vi "UDT_admittanceLibrary_selectData.vi"() -> (3 "Unit Test Framework Results":T1)   [LabVIEW 2017]
doc: "Use this template to create a user-defined test VI. Define your test requirements and wire the results to the <b>Result (Test)</b> control. Do not modify the <b>Unit Test Framework Results</b> indicator."
uses:
  <vilib>/utf/common/utf_test_result_troll.ctl
  <vilib>/utf/common/utf_test_result.ctl
  <vilib>/utf/common/utf_test_result_failure.ctl
  <vilib>/utf/common/utf_test_comparison_operators.ctl
  <vilib>/utf/common/utf_vi_tag.ctl
  RT/TypeDefs/allData.ctl
  RT/TypeDefs/dataOut.ctl
  RT/TypeDefs/dataIn.ctl
  <vilib>/Control Software Solutions Ltd/UTF Helper/SubVIs/UTF Double Equals.vi
  <vilib>/Control Software Solutions Ltd/UTF Helper/SubVIs/UTF Boolean Equals.vi
  RT/Admittance Controller/admittanceControllerLibrary.lvlib
  <vilib>/Control Software Solutions Ltd/UTF Helper/Unit Test Helper.lvlib
  <vilib>/utf/NI_UnitTestFramework.lvlib
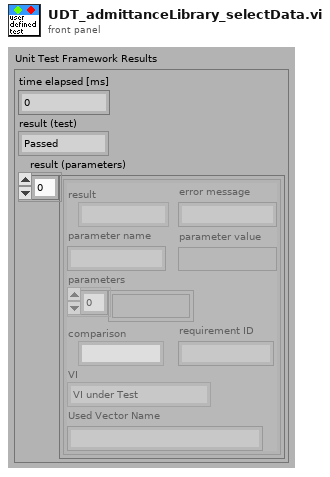
[diagram p1: front panel]
types:
  T1 = typedef "NI_UnitTestFramework.lvlib/utf_test_result_troll.ctl" = cluster{"time elapsed [ms]":u32, "result (test)":T2, "result (parameters)":T3[]}
  T2 = typedef "NI_UnitTestFramework.lvlib/utf_test_result.ctl" = enum16{"Passed", "Failed", "Error", "Skipped", "Not Processed"}
  T3 = typedef "NI_UnitTestFramework.lvlib/utf_test_result_failure.ctl" = cluster{"result":T2, "error message":string, "parameter name":string, "parameter value":variant, "parameters":variant[], "comparison":T4, "requirement ID":string, "VI":T5, "Used Vector Name":string}
  T4 = typedef "NI_UnitTestFramework.lvlib/utf_test_comparison_operators.ctl" = enum16{"=", "!=", ">", ">=", "<", "<=", "range", "symmetric tolerance", "asymmetric tolerance", "string contains", "string not contain", "array size", "string length", "array range", "by element", "array range (limit array)", "user-defined", "array contains", "array not contain", "vector length", "= (elm)", "!= (elm)", "= (case insensitive)", "!= (case insensitive)"}
  T5 = typedef "NI_UnitTestFramework.lvlib/utf_vi_tag.ctl" = enum16{"Setup VI", "VI under Test", "Teardown VI"}
  T6 = typedef "allData.ctl" = cluster{"DataOut":T7, "DataIn":T8}
  T7 = typedef "dataOut.ctl" = cluster{"X0pos":dbl, "Y0pos":dbl, "Z0pos":dbl, "Fx":dbl, "Fy":dbl, "Fz":dbl, "Encoder1":i32, "Encoder2":i32, "Pot1":dbl, "Pot2":dbl, "Theta0":dbl, "Theta1":dbl, "X1pos":dbl, "Y1pos":dbl, "Z1pos":dbl, "X2pos":dbl, "Y2pos":dbl, "Z2pos":dbl, "ErrorOccurred":bool}
  T8 = typedef "dataIn.ctl" = cluster{"Xtarget":dbl, "Ytarget":dbl, "Ztarget":dbl, "X_Attractor 1":dbl, "Y_Attractor 1":dbl, "Z_Attractor 1":dbl, "X_Attractor 2":dbl, "Y_Attractor 2":dbl, "Z_Attractor 2":dbl, "Traj Flag":bool, "DeadZone":dbl, "Assistance":bool, "Shutdown?":bool, "AssistanceLevel":dbl}
  T9 = typedef "admittanceControllerLibrary.lvlib/ControlVariables.ctl" = cluster{"ControlFlag":bool, "Fx":dbl, "Fy":dbl, "Theta0":dbl, "Theta1":dbl, "CurrentX":dbl, "CurrentY":dbl, "TargetX":dbl, "TargetY":dbl, "DeadZone":dbl, "Assistance?":bool, "AssitanceLevel":dbl}
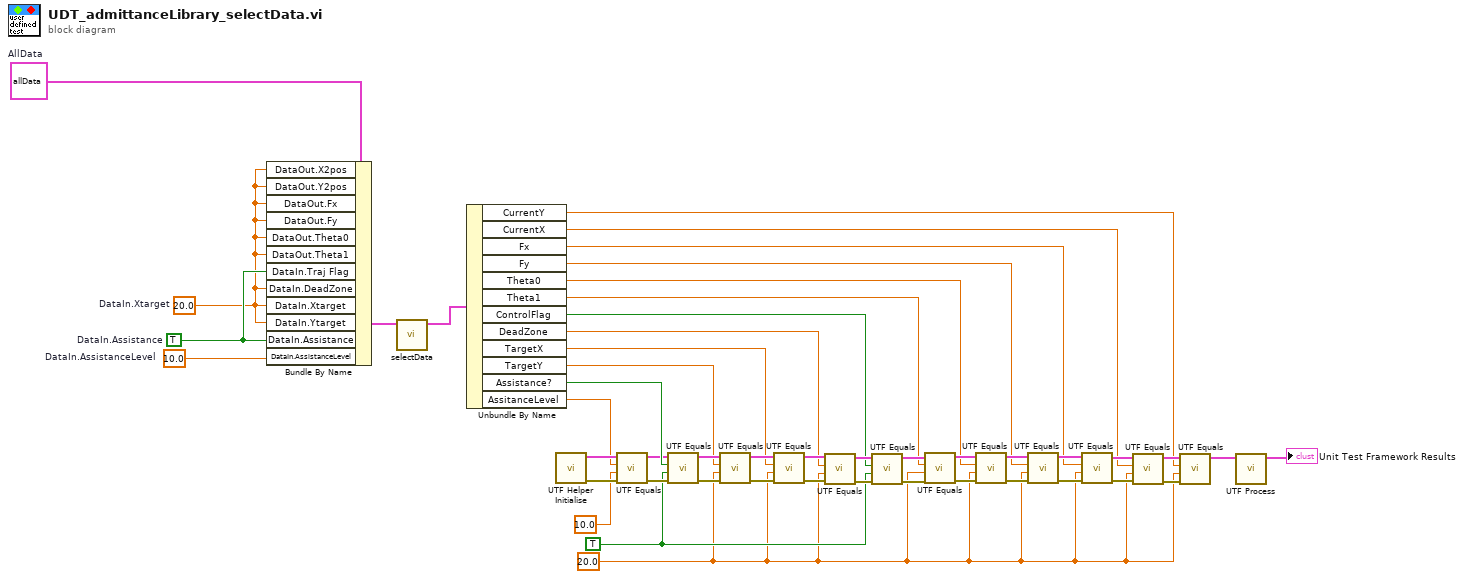
[diagram p0: block diagram]
diagram:
  w31 = 10.0  # DataIn.AssistanceLevel
  w7 = 20.0 ("DataIn.Xtarget")
  w23 = TRUE ("Test Value")
  w22 = TRUE  # DataIn.Assistance
  w21 = 20.0  # DataIn.Xtarget
  w47 = T6 {"DataOut"={"X0pos"=0.0, "Y0pos"=0.0, "Z0pos"=0.0, "Fx"=0.0, "Fy"=0.0, "Fz"=0.0, "Encoder1"=0, "Encoder2"=0, "Pot1"=0.0, "Pot2"=0.0, "Theta0"=0.0, "Theta1"=0.0, "X1pos"=0.0, "Y1pos"=0.0, "Z1pos"=0.0, "X2pos"=0.0, "Y2pos"=0.0, "Z2pos"=0.0, "ErrorOccurred"=FALSE}, "DataIn"={"Xtarget"=0.0, "Ytarget"=0.0, "Ztarget"=0.0, "X_Attractor 1"=0.0, "Y_Attractor 1"=0.0, "Z_Attractor 1"=0.0, "X_Attractor 2"=0.0, "Y_Attractor 2"=0.0, "Z_Attractor 2"=0.0, "Traj Flag"=FALSE, "DeadZone"=0.0, "Assistance"=FALSE, "Shutdown?"=FALSE, "AssistanceLevel"=0.0}}  # AllData
  n1 = Bundle By Name(cluster=w47, "DataOut.X2pos"=w21, "DataOut.Y2pos"=w21, "DataOut.Fx"=w21, "DataOut.Fy"=w21, "DataOut.Theta0"=w21, "DataOut.Theta1"=w21, "DataIn.Traj Flag"=w22, "DataIn.DeadZone"=w21, "DataIn.Xtarget"=w21, "DataIn.Ytarget"=w21, "DataIn.Assistance"=w22, "DataIn.AssistanceLevel"=w31) -> (w46:T6)
  n2 = call "selectData.vi"("AllData"=w46) -> (3:w45:T9)  [unwired: 9 in, 1 out]
  n3 = Unbundle By Name(w45) -> ("CurrentY"=w1:dbl, "CurrentX"=w2:dbl, "Fx"=w3:dbl, "Fy"=w4:dbl, "Theta0"=w5:dbl, "Theta1"=w6:dbl, "ControlFlag"=w24:bool, "DeadZone"=w27:dbl, "TargetX"=w37:dbl, "TargetY"=w38:dbl, "Assistance?"=w39:bool, "AssitanceLevel"=w32:dbl)
  n4 = call <vilib>:"UTF Helper Initialise.vi"() -> ("error out"=w33:errorcluster, "results array"=w34:T3[])  [unwired: 10 in]
  n5 = call-poly <vilib>:"UTF Equals.vi"("error in (no error)"=w33, "Test Value"=10.0 ("DataIn.Xtarget"), "Input"=w32, "Input Results"=w34) -> ("error out"=w36:errorcluster, "Output Results"=w35:T3[])  [unwired: 6 in]
  n6 = call-poly <vilib>:"UTF Equals.vi"("error in (no error)"=w36, "Test Value"=w23, "Input"=w39, "Input Results"=w35) -> ("error out"=w41:errorcluster, "Output Results"=w42:T3[])  [unwired: 6 in]
  n7 = call-poly <vilib>:"UTF Equals.vi"("error in (no error)"=w41, "Test Value"=w7, "Input"=w38, "Input Results"=w42) -> ("error out"=w40:errorcluster, "Output Results"=w43:T3[])  [unwired: 6 in]
  n8 = call-poly <vilib>:"UTF Equals.vi"("error in (no error)"=w40, "Test Value"=w7, "Input"=w37, "Input Results"=w43) -> ("error out"=w29:errorcluster, "Output Results"=w28:T3[])  [unwired: 6 in]
  n9 = call-poly <vilib>:"UTF Equals.vi"("error in (no error)"=w29, "Test Value"=w7, "Input"=w27, "Input Results"=w28) -> ("error out"=w26:errorcluster, "Output Results"=w25:T3[])  [unwired: 6 in]
  n10 = call-poly <vilib>:"UTF Equals.vi"("error in (no error)"=w26, "Test Value"=w23, "Input"=w24, "Input Results"=w25) -> ("error out"=w20:errorcluster, "Output Results"=w19:T3[])  [unwired: 6 in]
  n11 = call-poly <vilib>:"UTF Equals.vi"("error in (no error)"=w20, "Test Value"=w7, "Input"=w6, "Input Results"=w19) -> ("error out"=w18:errorcluster, "Output Results"=w9:T3[])  [unwired: 6 in]
  n12 = call-poly <vilib>:"UTF Equals.vi"("error in (no error)"=w18, "Test Value"=w7, "Input"=w5, "Input Results"=w9) -> ("error out"=w17:errorcluster, "Output Results"=w10:T3[])  [unwired: 6 in]
  n13 = call-poly <vilib>:"UTF Equals.vi"("error in (no error)"=w17, "Test Value"=w7, "Input"=w4, "Input Results"=w10) -> ("error out"=w16:errorcluster, "Output Results"=w11:T3[])  [unwired: 6 in]
  n14 = call-poly <vilib>:"UTF Equals.vi"("error in (no error)"=w16, "Test Value"=w7, "Input"=w3, "Input Results"=w11) -> ("error out"=w15:errorcluster, "Output Results"=w12:T3[])  [unwired: 6 in]
  n15 = call-poly <vilib>:"UTF Equals.vi"("error in (no error)"=w15, "Test Value"=w7, "Input"=w2, "Input Results"=w12) -> ("error out"=w14:errorcluster, "Output Results"=w13:T3[])  [unwired: 6 in]
  n16 = call-poly <vilib>:"UTF Equals.vi"("error in (no error)"=w14, "Test Value"=w7, "Input"=w1, "Input Results"=w13) -> ("Output Results"=w8:T3[])  [unwired: 6 in, 1 out]
  n17 = call <vilib>:"UTF Process.vi"("results array"=w8) -> ("Unit Test Framework Results"=→"Unit Test Framework Results":T1)  [unwired: 10 in]
